vi "setBiasVoltage.vi"(6 "Channel":u32, 8 "error in (no error)":errorcluster, 10 "Bias Voltage (V)":dbl, 11 "Instrument.VSource in":refnum<class "Instrument.VSource.lvclass">) -> (0 "error out":errorcluster, 3 "Instrument.VSource out":refnum<class "Instrument.VSource.lvclass">)   [LabVIEW 2019, in "Instrument.VSource.lvclass"]
uses:
  Instrument.VSource.lvclass
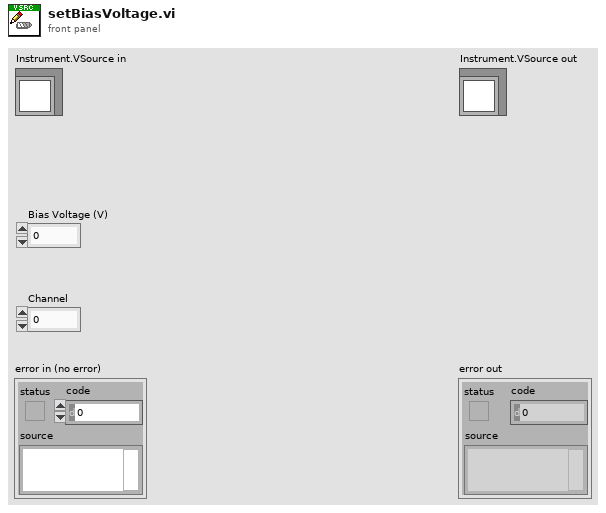
[diagram p1: front panel]
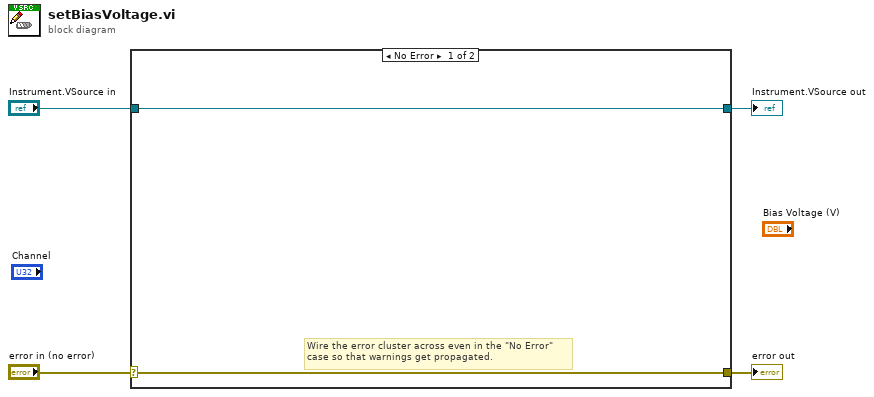
[diagram p0: block diagram]
diagram:
  n1 = case shown="No Error" "error in (no error)" {
    selector: "error in (no error)" -> [w5 w8]
    tunnel: [w5 w8] -> w3
    tunnel: [w6 w7] -> w1
    tunnel: "Instrument.VSource in" -> [w6 w7]
    frame No Error {
      # "Wire the error cluster across even in the \"No Error\"\ncase so that warnings get propagated."
    }
    frame Error {
    }
  }
  "error out" <- w3
  "Instrument.VSource out" <- w1
